vi "ChangeYourDisk.vi"() -> ()   [LabVIEW 2014]
panel:
  out "DiskTime":u32
  in  "Stop Button":bool
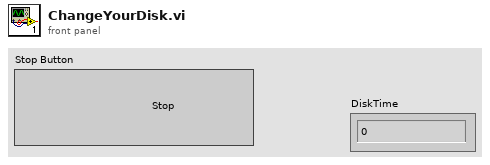
[diagram p1: front panel]
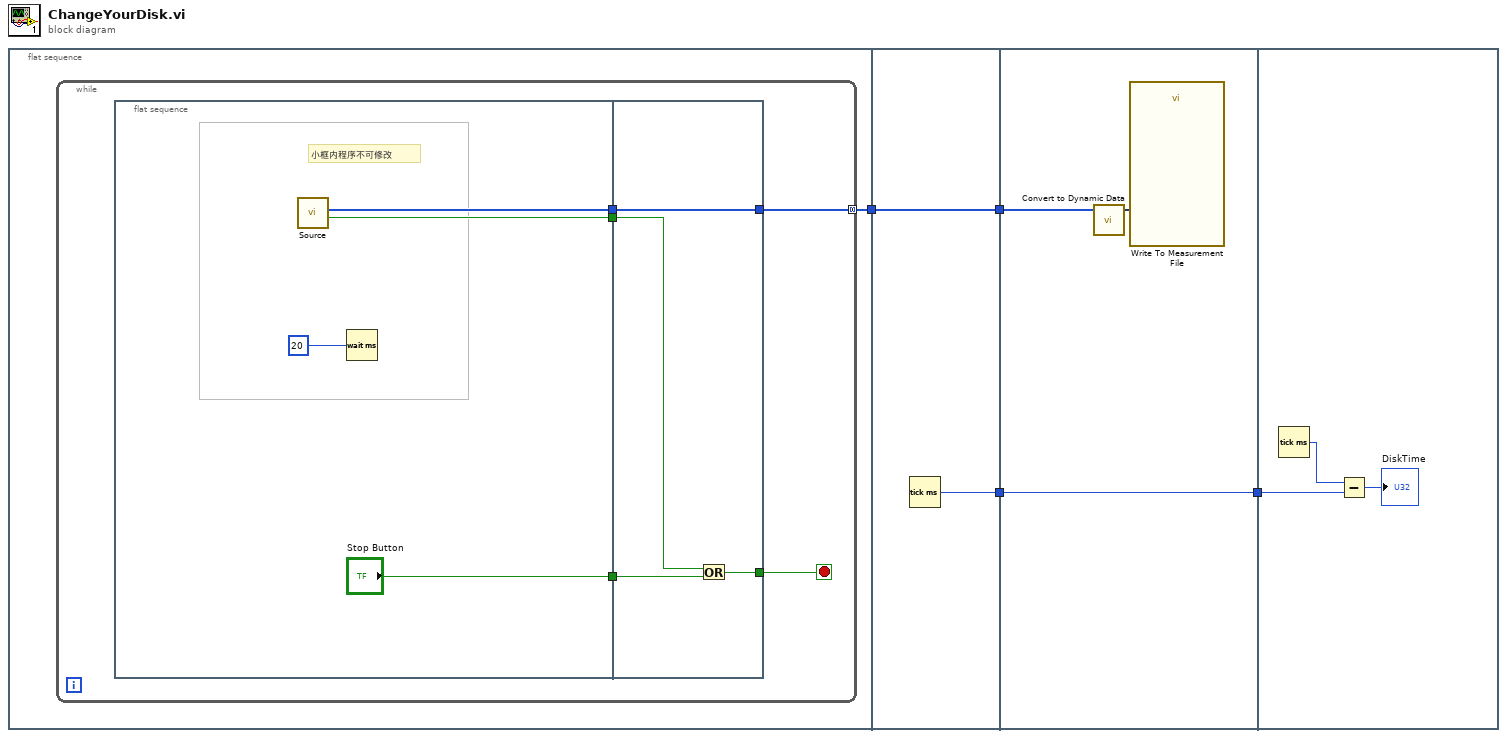
[diagram p0: block diagram]
diagram:
  n1 = flat-sequence {
    tunnel: [w5] -> w4
    tunnel: w4 -> [w20]
    tunnel: [w20] -> w3
    tunnel: [w19] -> w1
    tunnel: w3 -> [w22]
    tunnel: [w23] -> w2
    tunnel: w1 -> [w23]
    tunnel: w2 -> [w25]
    frame #0 {
      n2 = while {
        tunnel: [w10] -> w5 mode=concatenating
        stop <- w7 stop-if-true
        n3 = flat-sequence {
          tunnel: [w14] -> w9
          tunnel: ["Stop Button"] -> w8
          tunnel: [w12] -> w6
          tunnel: [w18] -> w10
          tunnel: w9 -> [w18]
          tunnel: w8 -> [w17]
          tunnel: [w16] -> w7
          tunnel: w6 -> [w15]
          frame #0 {
            # "小框内程序不可修改"
            n4 = call "Source.vi"() -> ("Terminate?"=w12:bool, "output"=w14:i16[])  [unwired: 2 in]
            n5 = Wait (ms)(milliseconds to wait=u32 20) -> ()  [unwired: 1 out]
          }
          frame #1 {
            n6 = Or(x=w15, y=w17) -> (x .or. y?=w16:bool)
          }
        }
      }
    }
    frame #1 {
      n7 = Tick Count (ms)() -> (millisecond timer value=w19:u32)
    }
    frame #2 {
      n8 = call "Convert to Dynamic Data"("Array"=w22) -> ("Dynamic Data Type"=w21:dynamicdata)  [unwired: 3 in]
      n9 = call "Write To Measurement File"("Signals"=w21) -> ()  [unwired: 16 in, 3 out]
    }
    frame #3 {
      n10 = Tick Count (ms)() -> (millisecond timer value=w26:u32)
      n11 = Subtract(x=w26, y=w25) -> (x-y=→"DiskTime":u32)
    }
  }
